vi "Configure_single_channel.vi"(8 "error in (no error)":errorcluster, 11 "Initialize_card in":refnum<class "Control_card.lvclass">) -> (0 "error out":errorcluster, 3 "Initialize_card out":refnum<class "Control_card.lvclass">)   [LabVIEW 2015, in "Control_card.lvclass"]
uses:
  Control_card.lvclass
panel:
  out "Error Code":u32
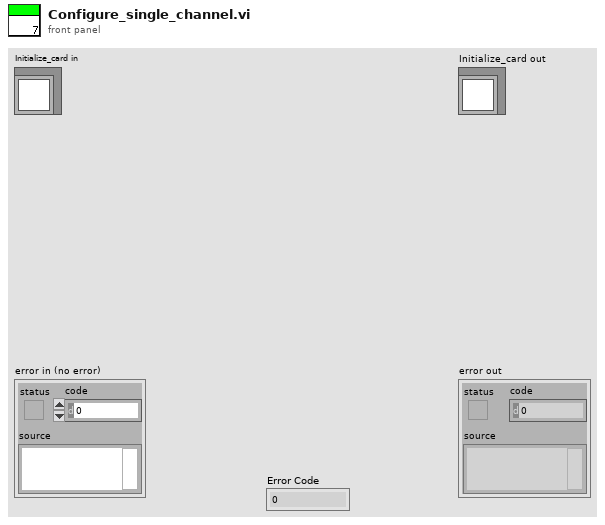
[diagram p1: front panel]
types:
  T1 = cluster{"Coupling":u16, "Differential Input":bool, "Direct-to-ADC":bool, "Range":u32, "Impedance":u32, "DC Offset":i32, "Filter":i32}
  T2 = cluster{"Handle":u32, "Sample size":u32, "Resolution":i32, "Offset":i32, "Channels":u32, "Boards":u32}
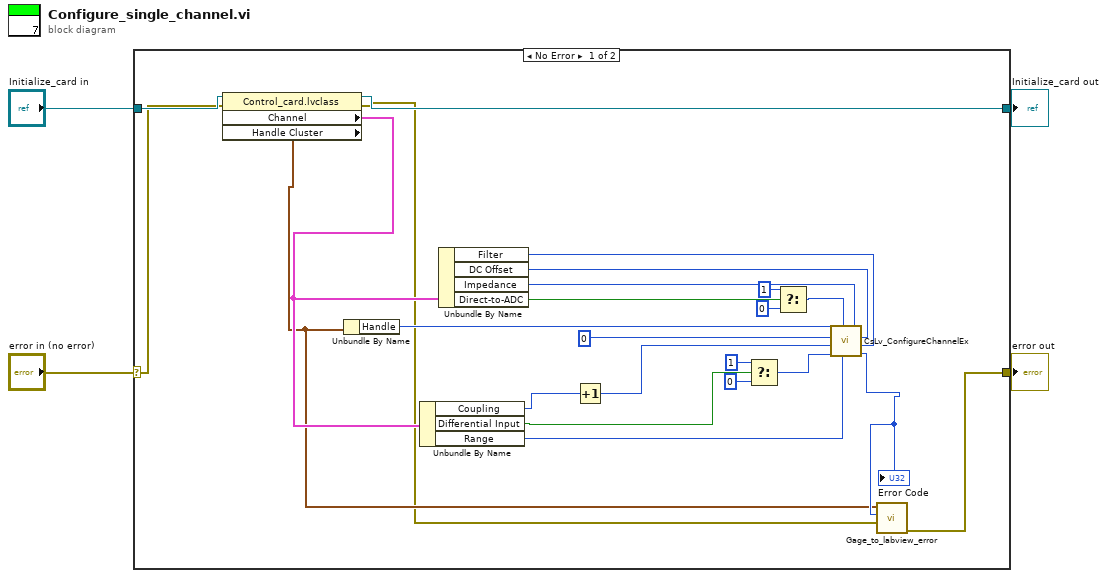
[diagram p0: block diagram]
diagram:
  n1 = case shown="No Error" "error in (no error)" {
    selector: "error in (no error)" -> [w26 w30]
    tunnel: [w5 w30] -> w3
    tunnel: [w27 w29] -> w1
    tunnel: "Initialize_card in" -> [w28 w29]
    frame No Error {
      n2 = property class="Control_card.lvclass"(reference=w28, error in=w26) -> (reference out=w27:refnum<class "Control_card.lvclass">, error out=w6:errorcluster, "Channel"=w12:T1, "Handle Cluster"=w7:T2)
      n3 = Unbundle By Name(w7) -> ("Handle"=w25:u32)
      n4 = Unbundle By Name(w12) -> ("Coupling"=w10:u16, "Differential Input"=w14:bool, "Range"=w13:u32)
      n5 = Unbundle By Name(w12) -> ("Filter"=w15:i32, "DC Offset"=w16:i32, "Impedance"=w17:u32, "Direct-to-ADC"=w18:bool)
      n6 = Increment(x=w10) -> (x+1=w9:u16)
      n7 = Select(t=u32 1, s=w14, f=0) -> (s? t:f=w21:u32)
      n8 = Select(t=1, s=w18, f=0) -> (s? t:f=w24:i32)
      n9 = call <userlib>:"CsLv_ConfigureChannelEx.vi"("Filter (0)"=w15, "DC Offset (0 mV)"=w16, "Impedance (1000000)"=w17, "Input range (2000 mV)"=w13, "Direct-to-ADC (0)"=w24, "Differential Input (0)"=w21, "Coupling (1)"=w9, "Channel (0)"=u32 0, "Handle"=w25) -> ("Error Code"=w8:i32)
      "Error Code" <- w8
      n10 = call "Gage_to_labview_error.vi"("Error In"=w6, "GaGe Error Number"=w8, "Handle Cluster"=w7) -> ("Error Out"=w5:errorcluster)  [unwired: 8 in]
    }
    frame Error {
    }
  }
  "error out" <- w3
  "Initialize_card out" <- w1
